vi "GetAllFolders.vi"(2 "error in (no error)":errorcluster, 3 "FolderPath":path) -> (0 "error out":errorcluster, 1 "Folders":string[](array[string]))   [LabVIEW 2013]
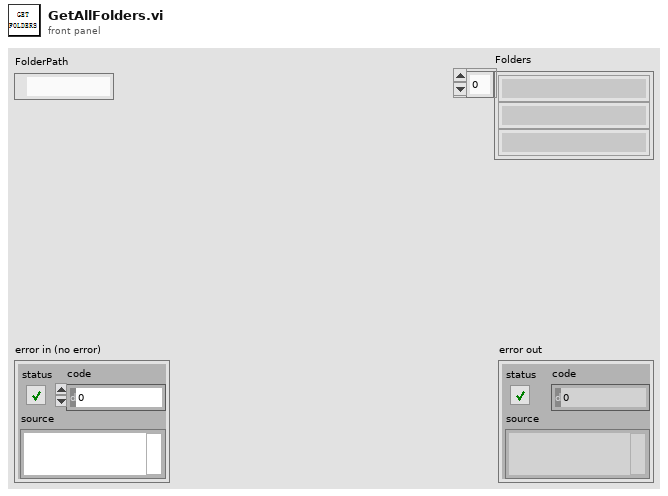
[diagram p1: front panel]
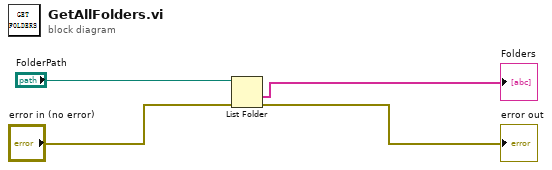
[diagram p0: block diagram]
diagram:
  n1 = List Folder(path="FolderPath", error in="error in (no error)") -> (folder names=→"Folders":string[], error out=→"error out":errorcluster)  [unwired: 2 in, 2 out]
